vi "rqcBob Get Detection Window.vi"(0 "rqcBob HW Control in":T1, 7 "PD.max meas length":u32, 11 "PD.detect fifo write enable":bool[](array[boolean])=[FALSE, FALSE]) -> (4 "rqcBob HW Control out":T1, 8 "window":u32, 15 "PD clicked":bool[](array[boolean]))   [LabVIEW 2018]
uses:
  Custom Controls/rqcBob HW Control.ctl
  <vilib>/RQC/FPGA Basic Logic/Counters/Counter (U32).vi
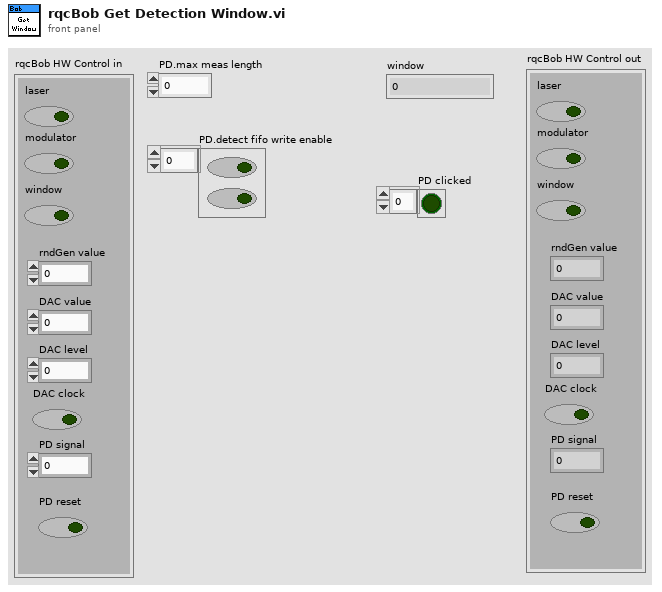
[diagram p1: front panel]
types:
  T1 = typedef "rqcBob HW Control.ctl" = cluster{"laser":bool, "modulator":bool, "window":bool, "rndGen value":u32, "DAC value":u16, "DAC level":u8, "DAC clock":bool, "PD signal":u8, "PD reset":bool}
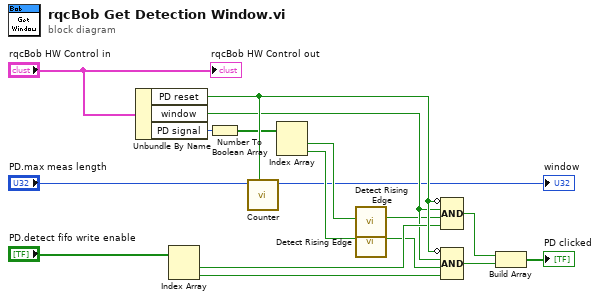
[diagram p0: block diagram]
diagram:
  n1 = Unbundle By Name("rqcBob HW Control in") -> ("PD reset"=w14:bool, "window"=w11:bool, "PD signal"=w10:u8)
  n2 = Index Array(array="PD.detect fifo write enable") -> (element #1=w13:bool, element #2=w12:bool)  [unwired: 2 in]
  n3 = Number To Boolean Array(number=w10) -> (Boolean array=w9:bool[])
  n4 = call-poly <vilib>:"Counter.vi"("reset"=w14, "bound"="PD.max meas length") -> ("count out"=→"window":u32)  [unwired: 8 in, 1 out]
  n5 = Index Array(array=w9) -> (element #1=w8:bool, element #2=w7:bool)  [unwired: 2 in]
  n6 = call <vilib>:"Detect Rising Edge.vi"("signal"=w8) -> ("edge detected"=w5:bool)  [unwired: 10 in]
  n7 = call <vilib>:"Detect Rising Edge.vi"("signal"=w7) -> ("edge detected"=w6:bool)  [unwired: 10 in]
  n8 = Compound Arithmetic op=AND(invert w14, w11, w5, w13) -> (w3:bool)
  n9 = Compound Arithmetic op=AND(invert w14, w11, w6, w12) -> (w2:bool)
  n10 = Build Array(w3, w2) -> (→"PD clicked":bool[])
  "rqcBob HW Control out" <- "rqcBob HW Control in"
